vi "plot_update_XY.vi"(0 "data":cluster{"X array":sgl[], " Y array":sgl[]} {"Y array" format="%.2f"; "X array" format="%.2f"}, 1 "data length":i32, 2 "x zoom factor":dbl format="%.2f", 3 "X range min":sgl format="%.2f", 4 "X range max":sgl format="%.2f", 5 "error in (no error)":errorcluster, 6 "graph ref":T1, 7 "X Scale.Name Label.Text":string, 8 "y range min":sgl format="%.2f", 9 "Y Scale.Name Label.Text":string, 10 "y range max":sgl format="%.2f", 11 "error rangeViolation":bool=TRUE, 12 "autoScale Y":bool, 13 "data idxStart":i32) -> (14 "dataVal max":sgl format="%.2f", 15 "dataVal min":sgl format="%.2f", 19 "error out":errorcluster)   [LabVIEW 2010, in "OSA.lvclass"]
doc: "Reads the contents of a <B>Thorlabs_OSA_64</B> object.\n\n[GOOP 1.0]"
uses:
  OSA.lvclass
  private/graph_intensity.ctl
panel:
  out "double precision float":dbl format="%^.4e"
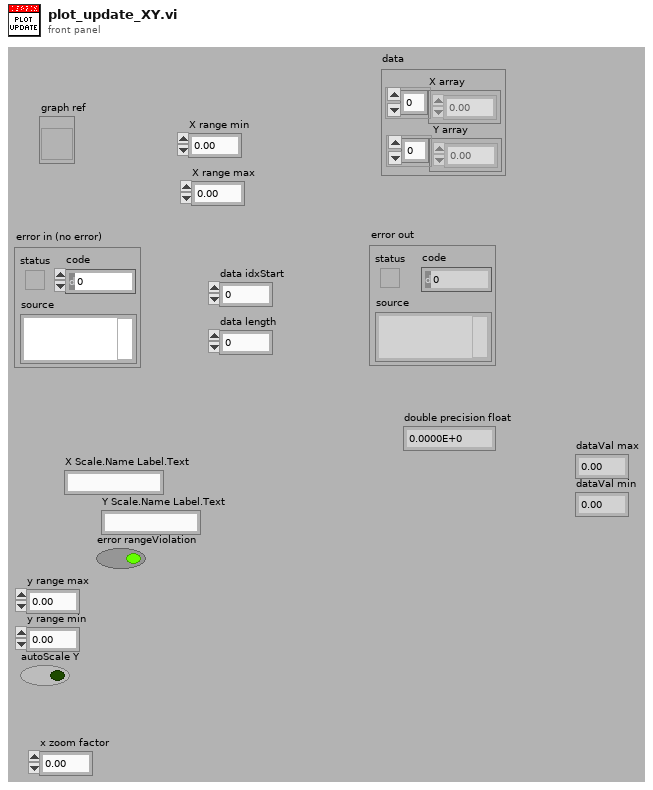
[diagram p1: front panel]
types:
  T1 = typedef "OSA.lvclass/graph_intensity.ctl" = refnum<vi>
  T2 = typedef "LVBoundsTypeDef.ctl" = cluster{"Width":u32, "Height":u32}
  T3 = cluster{"Name":string, "Color":u32, "Hair Style":u8, "Point Style":u8, "Name Visible":bool, "Trackable":bool, "Lock Style":u32, "Plot Number":u32, "Marker Index":i32, "Location":cluster{"X":dbl, "Y":dbl}}[]
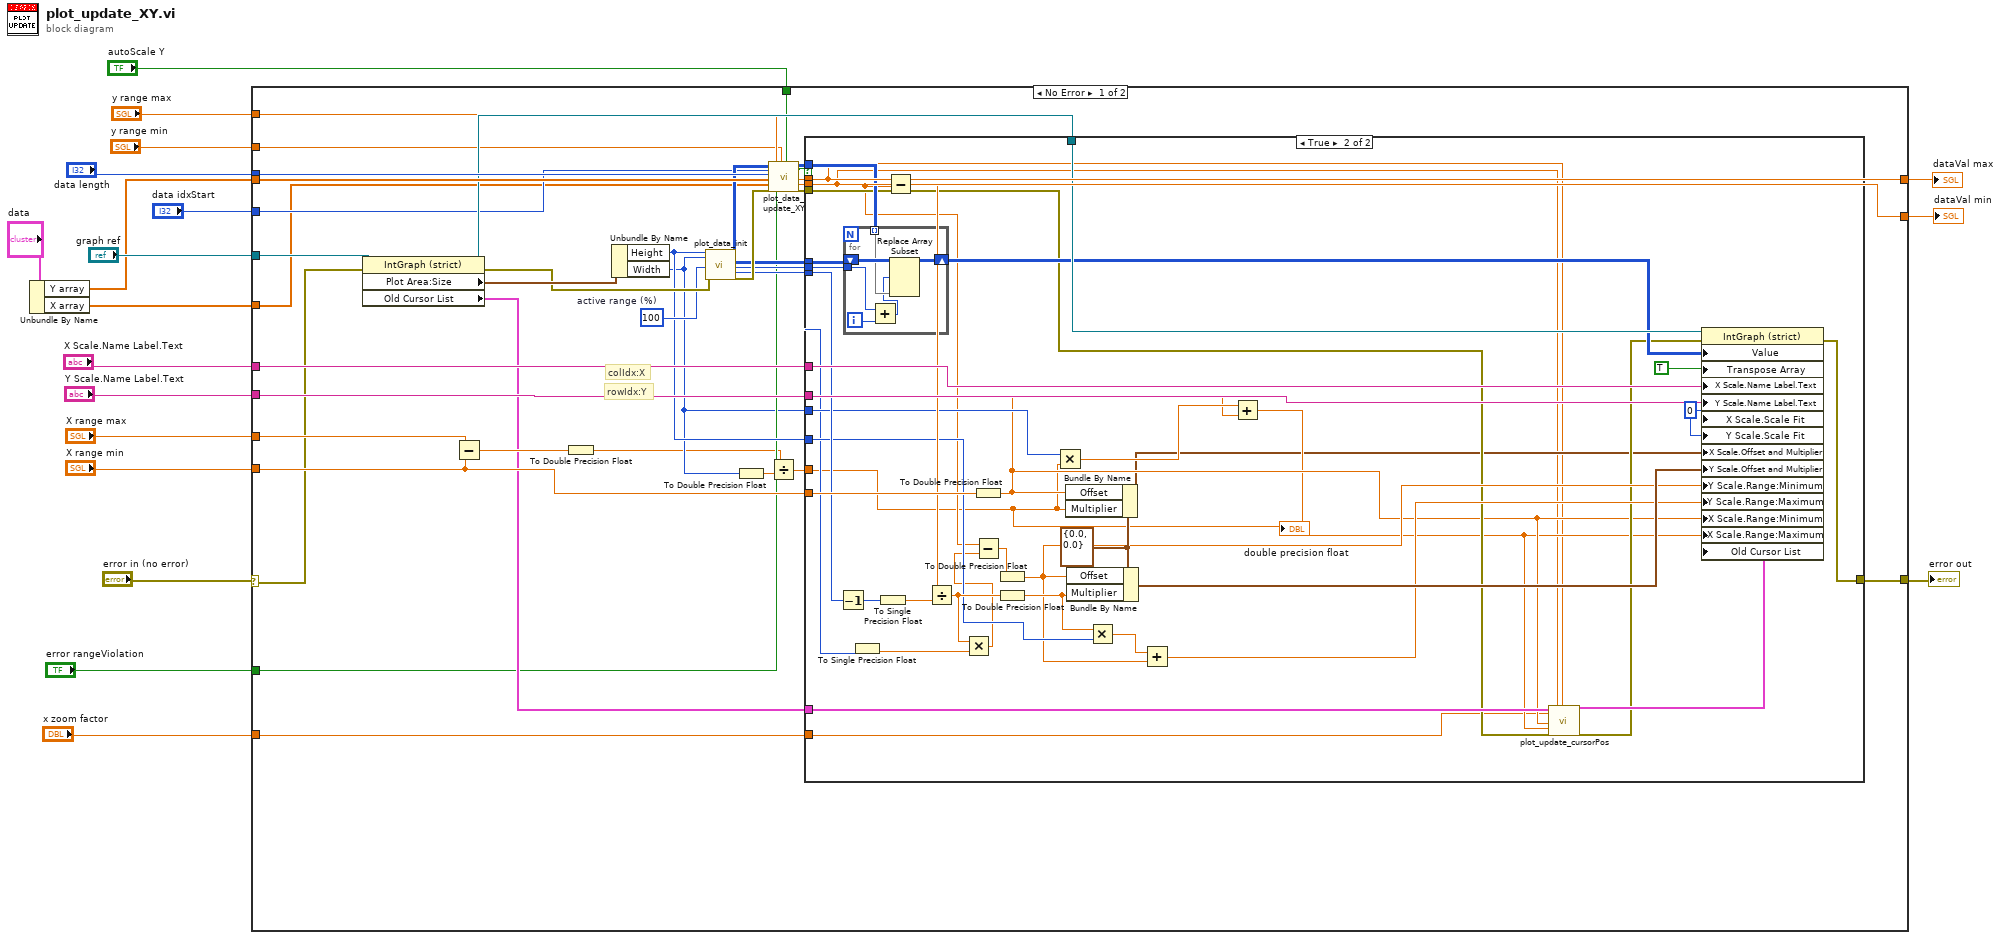
[diagram p0: block diagram]
diagram:
  n1 = Unbundle By Name("data") -> ("Y array"=w2:sgl[], "X array"=w1:sgl[])
  n2 = case shown="No Error" "error in (no error)" {
    selector: "error in (no error)" -> [w38 w105]
    tunnel: [w49 w105] -> w19
    tunnel: "graph ref" -> [w23 _]
    tunnel: "data length" -> [w53 _]
    tunnel: w2 -> [w52 _]
    tunnel: "X Scale.Name Label.Text" -> [w46 _]
    tunnel: "Y Scale.Name Label.Text" -> [w45 _]
    tunnel: "X range min" -> [w43 _]
    tunnel: "X range max" -> [w44 _]
    tunnel: "error rangeViolation" -> [w31 _]
    tunnel: "y range max" -> [w29 w104]
    tunnel: "y range min" -> [w28 w103]
    tunnel: "autoScale Y" -> [w27 _]
    tunnel: [w39 w104] -> w7
    tunnel: [w26 w103] -> w6
    tunnel: "x zoom factor" -> [w25 _]
    tunnel: "data idxStart" -> [w24 _]
    tunnel: w1 -> [w22 _]
    frame No Error {
      w51 = u32 100  # active range (%)
      # "colIdx:X"
      # "rowIdx:Y"
      # "Put your own code here"
      n3 = property class="IntGraph (strict)"(reference=w23, error in=w38) -> (reference out=w50:T1, error out=w55:errorcluster, "Plot Area:Size"=w56:T2, "Old Cursor List"=w33:T3)
      n4 = Subtract(x=w44, y=w43) -> (x-y=w42:sgl)
      n5 = To Double Precision Float(number=w42) -> (double precision float=w20:dbl)
      n6 = Unbundle By Name(w56) -> ("Height"=w35:u32, "Width"=w21:u32)
      n7 = call "plot_data_init.vi"("pixels Y"=w35, "pixels X"=w21, "active range (%)"=w51, "error in (no error)"=w55) -> ("plot data active"=w36:i32[][], "plot data"=w47:i32[][], "Y active idx start"=w34:i32, "Y active length"=w37:i32, "error out"=w54:errorcluster)  [unwired: 11 in]
      n8 = To Double Precision Float(number=w21) -> (double precision float=w41:dbl)
      n9 = call "plot_data_update_XY.vi"("plotData"=w36, "idx start"=w24, "length"=w53, "Y data"=w52, "X data"=w22, "error in (no error)"=w54, "max value Y"=w29, "error rangeViolation"=w31, "min value Y"=w28, "autoScale Y"=w27) -> ("plotData out"=w48:i32[][], "updated"=w30:bool, "dataVal max"=w39:sgl, "dataVal min"=w26:sgl, "error out"=w32:errorcluster)  [unwired: 2 in, 3 out]
      n10 = Divide(x=w20, y=w41) -> (x/y=w40:dbl)
      n11 = case shown="True" w30 {
        tunnel: w50 -> [_ w96]
        tunnel: [w57 w95] -> w49
        tunnel: w48 -> [_ w94]
        tunnel: w47 -> [_ w93]
        tunnel: w46 -> [_ w92]
        tunnel: w45 -> [_ w91]
        tunnel: w43 -> [_ w90]
        tunnel: w40 -> [_ w58]
        tunnel: w39 -> [_ w61]
        tunnel: w37 -> [_ w86]
        tunnel: w21 -> [_ w81]
        tunnel: w35 -> [_ w80]
        tunnel: w34 -> [_ w76]
        tunnel: w26 -> [_ w60]
        tunnel: w33 -> [_ w69]
        tunnel: w32 -> [w57 w67]
        tunnel: w25 -> [_ w59]
        frame False {
        }
        frame True {
          w62 = u8 0 ("X Scale.Scale Fit")
          w89 = cluster{"Offset":dbl, "Multiplier":dbl} {"Offset"=0.0, "Multiplier"=0.0} ("X Scale.Offset and Multiplier")
          n12 = Decrement(x=w86) -> (x-1=w73:i32)
          n13 = for {
            tunnel: w94 -> [w101] mode=indexing
            shift-right: [w100] -> w82
            shift-left: w93 -> [w102]
            tunnel: w76 -> [w98]
            i -> [w99]
            n14 = Add(x=w98, y=w99) -> (x+y=w97:i32)
            n15 = Replace Array Subset(array=w102, new element=w101, index (row)=w97) -> (w100:i32[][])  [unwired: 1 in]
          }
          n16 = To Single Precision Float(number=w76) -> (single precision float=w85:sgl)
          n17 = To Single Precision Float(number=w73) -> (single precision float=w84:sgl)
          n18 = Subtract(x=w61, y=w60) -> (x-y=w87:sgl)
          n19 = Divide(x=w87, y=w84) -> (x/y=w83:sgl)
          n20 = Multiply(x=w83, y=w85) -> (x*y=w75:sgl)
          n21 = To Double Precision Float(number=w90) -> (double precision float=w65:dbl)
          n22 = Subtract(x=w60, y=w75) -> (x-y=w74:sgl)
          n23 = To Double Precision Float(number=w74) -> (double precision float=w72:dbl)
          n24 = To Double Precision Float(number=w83) -> (double precision float=w77:dbl)
          n25 = Multiply(x=w81, y=w58) -> (x*y=w78:dbl)
          n26 = Bundle By Name(cluster=w89, "Offset"=w65, "Multiplier"=w58) -> (w63:cluster{"Offset":dbl, "Multiplier":dbl})
          n27 = Bundle By Name(cluster=w89, "Offset"=w72, "Multiplier"=w77) -> (w88:cluster{"Offset":dbl, "Multiplier":dbl})
          n28 = Multiply(x=w77, y=w80) -> (x*y=w79:dbl)
          n29 = Add(x=w79, y=w72) -> (x+y=w71:dbl)
          n30 = Add(x=w78, y=w65) -> (x+y=w64:dbl)
          n31 = call "plot_update_cursorPos.vi"("cursor list"=w69, "x zoom factor"=w59, "x min"=w65, "x max"=w64, "error in (no error)"=w67, "y max"=w60, "y min"=w61) -> ("cursor list out"=w68:T3, "error out"=w66:errorcluster)  [unwired: 11 in]
          n32 = property class="IntGraph (strict)"(reference=w96, error in=w66, "Value"=w82, "Transpose Array"=TRUE, "X Scale.Name Label.Text"=w92, "Y Scale.Name Label.Text"=w91, "X Scale.Scale Fit"=w62, "Y Scale.Scale Fit"=w62, "X Scale.Offset and Multiplier"=w63, "Y Scale.Offset and Multiplier"=w88, "Y Scale.Range:Minimum"=w72, "Y Scale.Range:Maximum"=w71, "X Scale.Range:Minimum"=w65, "X Scale.Range:Maximum"=w64, "Old Cursor List"=w68) -> (error out=w95:errorcluster)  [unwired: 1 out]
          "double precision float" <- w58
        }
      }
    }
    frame Error {
      # "Error"
    }
  }
  "error out" <- w19
  "dataVal max" <- w7
  "dataVal min" <- w6
